vi "Get Write Setup.vi"(8 "error in (no error)":errorcluster, 11 "RxTx in":refnum<class "RxTx.lvclass">) -> (0 "error out":errorcluster, 3 "RxTx out":refnum<class "RxTx.lvclass">)   [LabVIEW 2018, in "RxTx.lvclass"]
uses:
  RxTx.lvclass
  RxTx.lvclass/RxTx.ctl
  Interface/Interface.lvclass
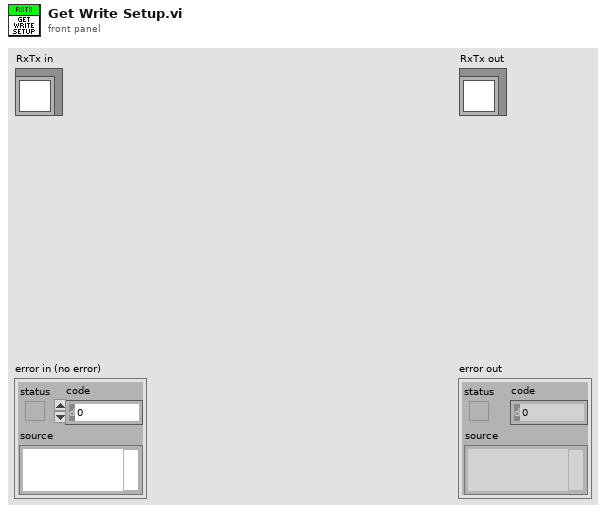
[diagram p1: front panel]
types:
  T1 = cluster{"PREAMP":u16, "READOUT_RATE":u16, "EM_GAIN":u16, "VBIN":u16, "INITIAL_LINE":u16, "INITIAL_COLUMN":u16, "FINAL_LINE":u16, "FINAL_COLUMN":u16, "TRIGGER_MODE":u16, "HBIN":u16, "SHUTTER_TTL":u16, "SHUTTER_MODE":u16, "SHUTTER_OPENING_TIME":u16, "SHUTTER_CLOSING_TIME":u16, "VERTICAL_SHIFT_SPEED":u16, "READ_MODE":u16, "FRAME_TRANSFER":bool, "VERTICAL_CLOCK_VOLTAGE":u16, "ACQUISITION_MODE":u16, "AD_CHANNEL":u16, "EM_MODE":u16}
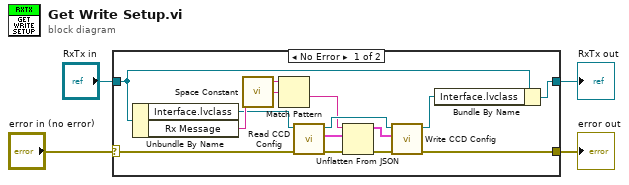
[diagram p0: block diagram]
diagram:
  n1 = case shown="No Error" "error in (no error)" {
    selector: "error in (no error)" -> [w13 w20]
    tunnel: [w12 w20] -> w2
    tunnel: [w15 w19] -> w1
    tunnel: "RxTx in" -> [w16 w19]
    frame No Error {
      n2 = Unbundle By Name(w16) -> ("Interface.lvclass"=w14:refnum<class "Interface.lvclass">, "Rx Message"=w17:string)
      n3 = call <vilib>:"Space Constant.vi"() -> ("String"=w18:string)
      n4 = Match Pattern(string=w17, regular expression=w18) -> (after substring=w6:string)  [unwired: 1 in, 3 out]
      n5 = call "Read CCD Config.vi"("error in (no error)"=w13, "Interface in"=w14) -> ("error out"=w8:errorcluster, "Previous CCD Config"=w7:T1, "Interface out"=w10:refnum<class "Interface.lvclass">)  [unwired: 7 in]
      n6 = Unflatten From JSON(JSON string=w6, type and defaults=w7, error in (no error)=w8) -> (value=w5:T1, error out=w9:errorcluster)  [unwired: 4 in]
      n7 = call "Write CCD Config.vi"("error in (no error)"=w9, "CCD Config"=w5, "Interface in"=w10) -> ("error out"=w12:errorcluster, "Interface out"=w11:refnum<class "Interface.lvclass">)  [unwired: 7 in]
      n8 = Bundle By Name(cluster=w16, "Interface.lvclass"=w11) -> (w15:refnum<class "RxTx.lvclass">)
    }
    frame Error {
    }
  }
  "error out" <- w2
  "RxTx out" <- w1
